vi "Flex Msg Populate and Override.vi"(8 "error in (no error)":errorcluster, 9 "Sequence Element":T1, 10 "Override Look up table in":variant, 11 "Flex Msg in":refnum<class "Flex Msg.lvclass">) -> (0 "error out":errorcluster, 1 "Flex Data Elements Cluster Array":T4, 2 "Override Look up table out":variant, 3 "Flex Msg out":refnum<class "Flex Msg.lvclass">)   [LabVIEW 2020, in "Sequencer.lvlib"]
doc: "Populate the Flex Msg with the configured data and override when requested. Also return array override data in 'Flex Data Elements Cluster Array'."
uses:
  Sequencer.lvlib
  PPL/HDH.Actor Framework.Core.Msg.lvlibp/Flex Msg/Flex Msg.lvclass
  Controls/Ctl_FlexDataElements.ctl
  Controls/Ctl_FlexDataElement.ctl
  Controls/Ctl_SequenceElement.ctl
  Controls/Ctl_SequenceControlElement.ctl
  PPL/HDH.Actor Framework.Core.Msg.lvlibp/Flex Msg/Controls/Ctl_Control Element.ctl
  PPL/HDH.Actor Framework.Core.Msg.lvlibp/Flex Msg/Data Access Handlers/Set Controls/Set Controls.lvclass
  C:/Current projects/WS/PPL/HDH.Actor Framework.Core.Msg.lvlibp/Flex Msg/Data Access Handlers/Data Access Handler/Data Access Handler.lvclass
  PPL/HDH.Actor Framework.Core.Msg.lvlibp
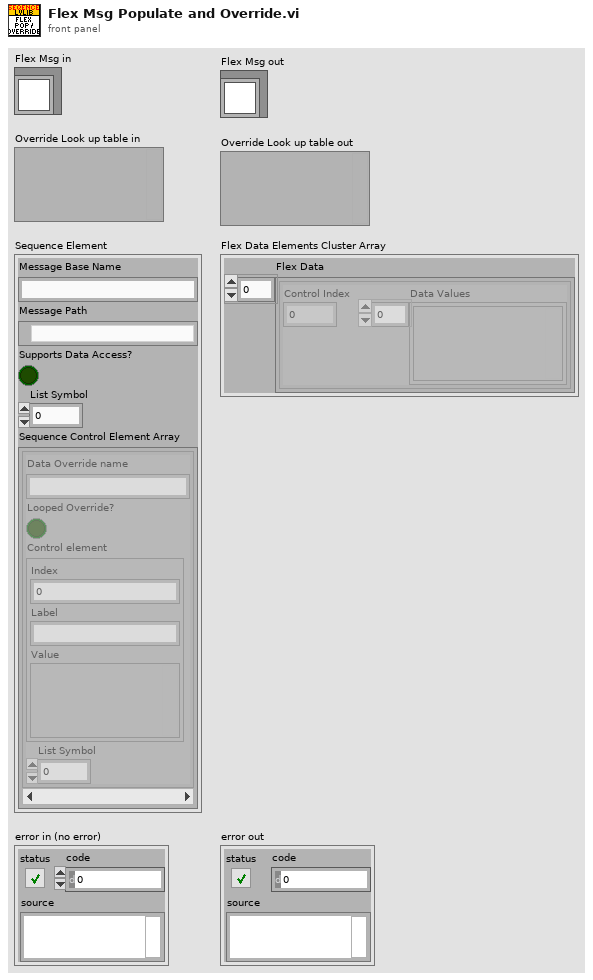
[diagram p1: front panel]
types:
  T1 = typedef "Sequencer.lvlib/Ctl_SequenceElement.ctl" = cluster{"Message Base Name":string, "Message Path":path, "Supports Data Access?":bool, "List Symbol":i32, "Sequence Control Element Array":T2[]}
  T2 = typedef "Sequencer.lvlib/Ctl_SequenceControlElement.ctl" = cluster{"Data Override name":string, "Looped Override?":bool, "Control element":T3, "List Symbol":i32}
  T3 = typedef "HDH.Actor Framework.Core.Msg.lvlibp/Ctl_Control Element.ctl" = cluster{"Index":i32, "Label":string, "Value":variant}
  T4 = typedef "Sequencer.lvlib/Ctl_FlexDataElements.ctl" = cluster{"Flex Data":T5[]}
  T5 = typedef "Sequencer.lvlib/Ctl_FlexDataElement.ctl" = cluster{"Control Index":i32, "Data Values":variant[]}
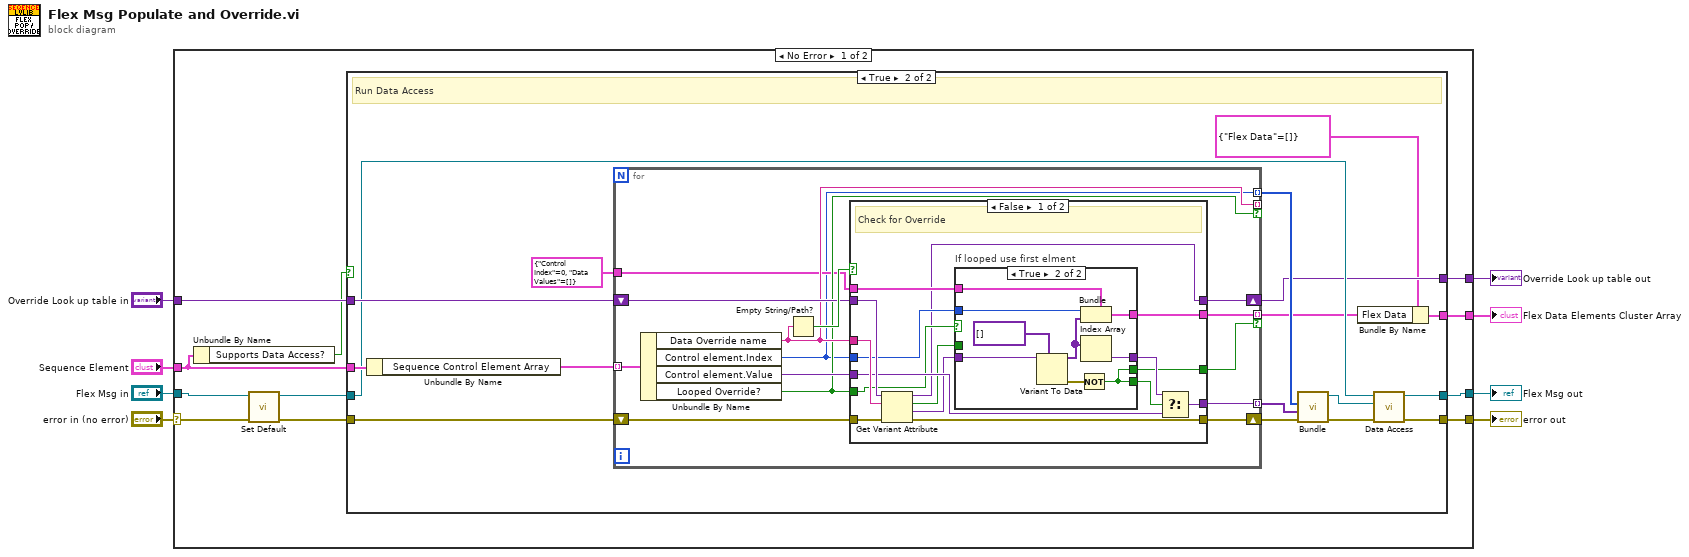
[diagram p0: block diagram]
diagram:
  n1 = case shown="No Error" "error in (no error)" {
    selector: "error in (no error)" -> [w14 w87]
    tunnel: [w19 w88] -> w8
    tunnel: [w18 w87] -> w7
    tunnel: [w17 w89] -> w6
    tunnel: [w16 _] -> w5
    tunnel: "Flex Msg in" -> [w12 w88]
    tunnel: "Override Look up table in" -> [w11 w89]
    tunnel: "Sequence Element" -> [w10 _]
    frame No Error {
      n2 = Unbundle By Name(w10) -> ("Supports Data Access?"=w9:bool)
      n3 = call-dynamic "Set Default.vi"("error in (no error)"=w14, "Flex Msg in"=w12) -> ("error out"=w15:errorcluster, "Flex Msg out"=w13:refnum<class "Flex Msg.lvclass">)  [unwired: 8 in]
      n4 = case shown="True" w9 {
        tunnel: [w22 w27] -> w19
        tunnel: w13 -> [w22 w32]
        tunnel: [w21 w26] -> w18
        tunnel: w15 -> [w21 w36]
        tunnel: w10 -> [_ w39]
        tunnel: w11 -> [w20 w37]
        tunnel: [_ w28] -> w16
        tunnel: [w20 w25] -> w17
        frame False {
          # "No data Access support"
        }
        frame True {
          # "Run Data Access"
          n5 = Unbundle By Name(w39) -> ("Sequence Control Element Array"=w38:T2[])
          n6 = for {
            tunnel: w38 -> [w53] mode=indexing
            tunnel: [w43] -> w35 mode=indexing
            tunnel: [w49] -> w34 mode=indexing
            shift-right: [w47] -> w33
            shift-left: w36 -> [w48]
            tunnel: [w46] -> _ mode=indexing if=w45
            tunnel: T5 {"Control Index"=0, "Data Values"=[]} ("Flex Data Element") -> [w44]
            tunnel: [w42] -> w29 mode=indexing if=w41
            shift-right: [w40] -> w25
            shift-left: w37 -> [w51]
            n7 = Unbundle By Name(w53) -> ("Data Override name"=w46:string, "Control element.Index"=w43:i32, "Control element.Value"=w50:variant, "Looped Override?"=w45:bool)
            n8 = Empty String/Path?(string/path=w46) -> (empty?=w52:bool)
            n9 = case shown="False" w52 {
              tunnel: w51 -> [w69 w83]
              tunnel: w46 -> [w68 _]
              tunnel: w50 -> [w67 w86]
              tunnel: [w66 w86] -> w49
              tunnel: w48 -> [w65 w85]
              tunnel: [w59 w85] -> w47
              tunnel: w45 -> [w64 _]
              tunnel: w44 -> [w58 w84]
              tunnel: w43 -> [w57 _]
              tunnel: [w56 w84] -> w42
              tunnel: [w55 _] -> w41
              tunnel: [w54 w83] -> w40
              frame False {
                # "Check for Override"
                n10 = Get Variant Attribute(Variant=w69, name=w68, error in=w65) -> (duplicate Variant=w54:variant, found=w60:bool, value=w62:variant, error out=w59:errorcluster)  [unwired: 1 in]
                n11 = case "If looped use first elment" shown="True" w64 {
                  selector: w64 -> [w70 _]
                  tunnel: [w73 w80] -> w63
                  tunnel: w62 -> [w73 w82]
                  tunnel: [w72 w74] -> w61
                  tunnel: w60 -> [w72 _]
                  tunnel: w58 -> [w71 w78]
                  tunnel: [w71 w75] -> w56
                  tunnel: w57 -> [_ w77]
                  tunnel: [w70 w74] -> w55
                  frame False {
                  }
                  frame True {
                    n12 = Variant To Data(type=variant[] [], Variant=w82) -> (data=w76:variant[], error out=w79:errorcluster)  [unwired: 1 in]
                    n13 = Not(x=w79) -> (.not. x?=w74:bool)
                    n14 = Bundle(cluster=w78, "Control Index"=w77, "Data Values"=w76) -> (w75:T5)
                    n15 = Index Array(array=w76) -> (element=w80:variant)  [unwired: 1 in]
                  }
                }
                n16 = Select(t=w63, s=w61, f=w67) -> (s? t:f=w66:variant)
              }
              frame True {
                # "No Override"
              }
            }
          }
          n17 = call "Bundle.vi"("error in (no error)"=w33, "Data Values"=w34, "Control Indices"=w35) -> ("error out"=w30:errorcluster, "Set Controls out"=w31:refnum<class "Set Controls.lvclass">)  [unwired: 7 in]
          n18 = Bundle By Name(cluster=T4 {"Flex Data"=[]} ("Flex Data Elements Cluster Array"), "Flex Data"=w29) -> (w28:T4)
          n19 = call-dynamic "Data Access.vi"("error in (no error)"=w30, "Data Access Handler"=w31, "Flex Msg in"=w32) -> ("error out"=w26:errorcluster, "Flex Msg out"=w27:refnum<class "Flex Msg.lvclass">)  [unwired: 7 in]
        }
      }
    }
    frame Error {
    }
  }
  "Flex Msg out" <- w8
  "error out" <- w7
  "Override Look up table out" <- w6
  "Flex Data Elements Cluster Array" <- w5
